vi "Fit btk.vi"() -> ()   [LabVIEW 2021]
uses:
  Parameters.ctl
panel:
  in  "Scale":dbl
  in  "Parameters":T1={"Gama"=0.001, "Delta"=0.03, "Z"=1.0, "P"=0.0, "T"=50.0, "Lower limit"=-10.0, "Upper limit"=10.0, "Resolution"=0.01}
  out "x/y":dbl format="%#_6p"
  in  "Max current":dbl format="%#_6p"
  in  "Resistance in series":dbl=30.0
  out "XY Graph":cluster{dbl[], dbl[]}[](graph)
  out "group/channel names":string[][](array[string])
  out "group names":string[](array[string])
  in  "File Path":path
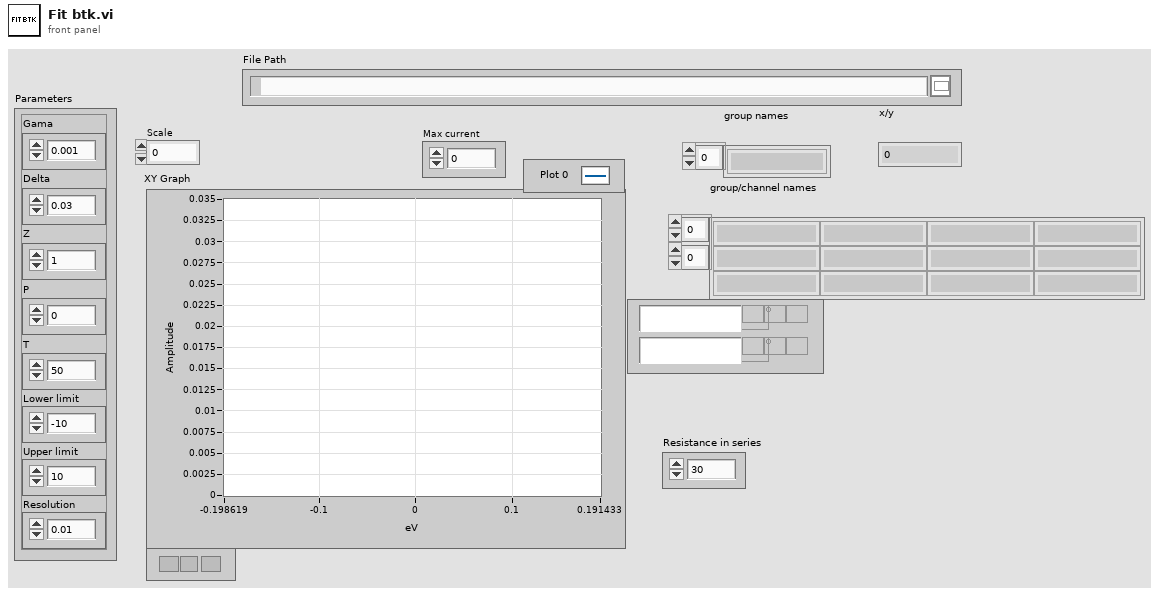
[diagram p1: front panel]
types:
  T1 = typedef "Parameters.ctl" = cluster{"Gama":dbl, "Delta":dbl, "Z":dbl, "P":dbl, "T":dbl, "Lower limit":dbl, "Upper limit":dbl, "Resolution":dbl}
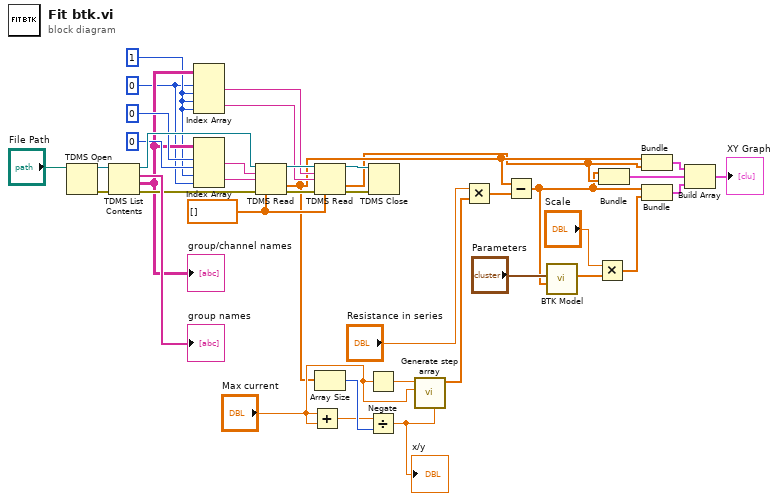
[diagram p0: block diagram]
diagram:
  w21 = dbl[] []
  w20 = 1 ("disabled index (col)")
  w19 = 0 ("index (row)")
  n1 = TDMS Open(11:"File Path") -> (0:w38:errorcluster, 3:w37:refnum<k34>)  [unwired: 6 in]
  n2 = TDMS List Contents(4:w38, 7:w37) -> (0:w34:errorcluster, 1:w31:string[][], 2:→"group names":string[], 3:w35:refnum<k34>)  [unwired: 1 in]
  "group/channel names" <- w31
  n3 = Index Array(array=w31, index (row) #1=w19, index (col) #1=w20, index (row) #2=w20, index (col) #2=w20) -> (element #1=w26:string, element #2=w25:string)
  n4 = Index Array(array=w31, index (row) #1=0 ("index (row)"), index (col) #1=0 ("disabled index (col)"), index (row) #2=w20, index (col) #2=w19) -> (element #1=w28:string, element #2=w27:string)
  n5 = TDMS Read(0:w35, 5:w28, 7:w27, 11:w34, 12:w21) -> (4:w29:refnum<k34>, 10:w9:dbl[], 15:w30:errorcluster)  [unwired: 3 in, 3 out]
  n6 = Add(x="Max current", y="Max current") -> (x+y=w16:dbl)
  n7 = TDMS Read(0:w29, 5:w26, 7:w25, 11:w30, 12:w21) -> (4:w23:refnum<k34>, 10:w8:dbl[], 15:w24:errorcluster)  [unwired: 3 in, 3 out]
  n8 = Array Size(array=w9) -> (size(s)=w17:i32)
  n9 = Negate(x="Max current") -> (-x=w18:dbl)
  n10 = Divide(x=w16, y=w17) -> (x/y=w14:dbl)
  "x/y" <- w14
  n11 = TDMS Close(8:w24, 11:w23) -> ()  [unwired: 2 out]
  n12 = call "Generate step array.vi"("Step"=w14, "End"="Max current", "Start"=w18) -> ("Steps"=w12:dbl[])  [unwired: 8 in]
  n13 = Multiply(x="Resistance in series", y=w12) -> (x*y=w11:dbl[])
  n14 = Subtract(x=w9, y=w11) -> (x-y=w5:dbl[])
  n15 = call "BTK Model.vi"("V"=w5, "Parameters"="Parameters") -> ("Conductivity"=w4:dbl[])  [unwired: 9 in]
  n16 = Multiply(x="Scale", y=w4) -> (x*y=w2:dbl[])
  n17 = Bundle(w5, w8) -> (w7:cluster{dbl[], dbl[]})  [unwired: 1 in]
  n18 = Bundle(w9, w8) -> (w22:cluster{dbl[], dbl[]})  [unwired: 1 in]
  n19 = Bundle(w5, w2) -> (w3:cluster{dbl[], dbl[]})  [unwired: 1 in]
  n20 = Build Array(w22, w7, w3) -> (→"XY Graph":cluster{dbl[], dbl[]}[])
